vi "DE_Compare Population.vi"(10 "Population B":T2, 11 "Population A":T2) -> (2 "feasible?":bool, 3 "population comparison":T1 items=["A dominates B", "B dominates A", "Neither dominates", "A = B"])   [LabVIEW 2020, in "NI_AAL_GlobalOptimization.lvlib"]
uses:
  <vilib>/gmath/NI_AAL_GlobalOptimization.lvlib
  <vilib>/gmath/GlobalOptimization.llb/DE_Population.ctl
  <vilib>/gmath/GlobalOptimization.llb/DE_Population Comparison.ctl
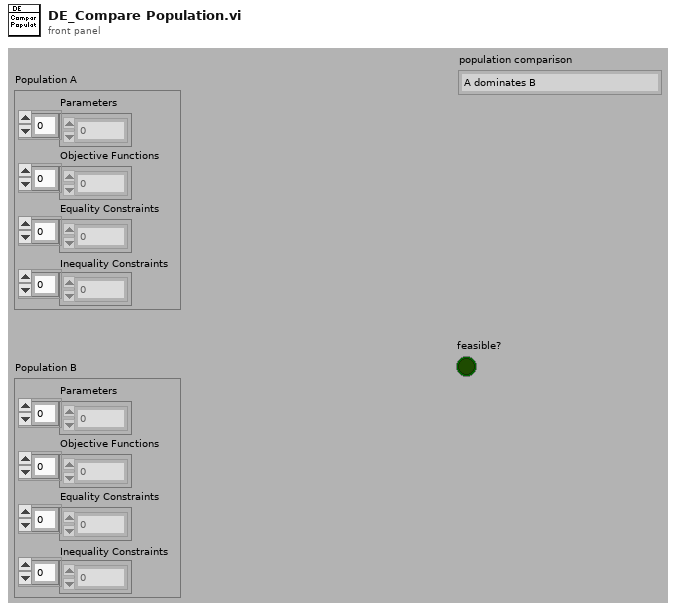
[diagram p1: front panel]
types:
  T1 = typedef "NI_AAL_GlobalOptimization.lvlib/DE_Population Comparison.ctl" = u16
  T2 = typedef "NI_AAL_GlobalOptimization.lvlib/DE_Population.ctl" = cluster{"Parameters":dbl[], "Objective Functions":dbl[], "Equality Constraints":dbl[], "Inequality Constraints":dbl[]}
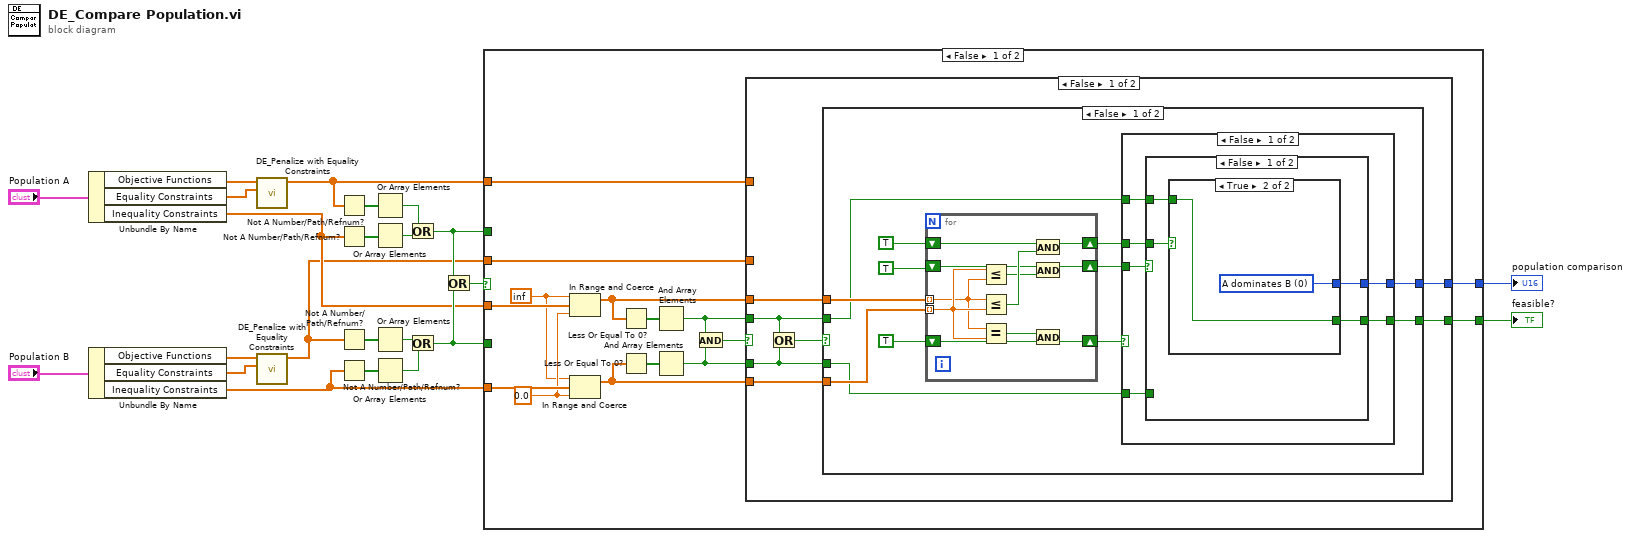
[diagram p0: block diagram]
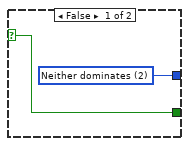
[diagram p2: hidden frame]
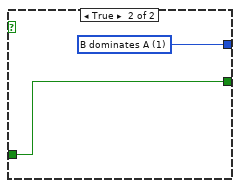
[diagram p3: hidden frame]
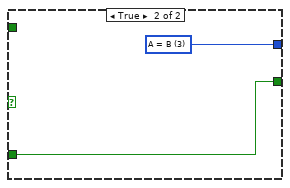
[diagram p4: hidden frame]
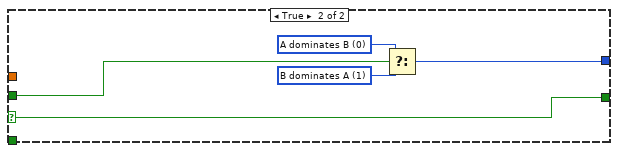
[diagram p5: hidden frame]
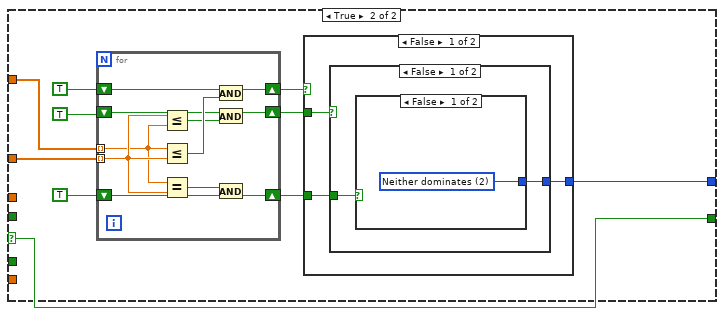
[diagram p6: hidden frame]
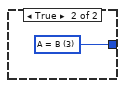
[diagram p7: hidden frame]
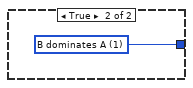
[diagram p8: hidden frame]
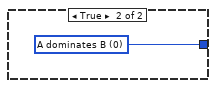
[diagram p9: hidden frame]
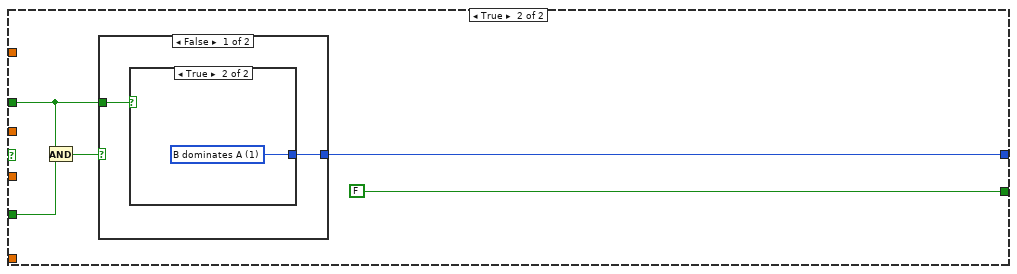
[diagram p10: hidden frame]
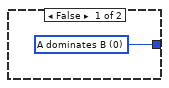
[diagram p11: hidden frame]
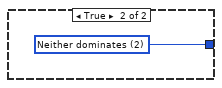
[diagram p12: hidden frame]
diagram:
  n1 = Unbundle By Name("Population A") -> ("Objective Functions"=w6:dbl[], "Equality Constraints"=w7:dbl[], "Inequality Constraints"=w8:dbl[])
  n2 = Unbundle By Name("Population B") -> ("Objective Functions"=w2:dbl[], "Equality Constraints"=w3:dbl[], "Inequality Constraints"=w4:dbl[])
  n3 = call <vilib>:"DE_Penalize with Equality Constraints.vi"("Equality Constraints"=w7, "Objective Functions In"=w6) -> ("Objective Functions Out"=w5:dbl[])  [unwired: 9 in]
  n4 = call <vilib>:"DE_Penalize with Equality Constraints.vi"("Equality Constraints"=w3, "Objective Functions In"=w2) -> ("Objective Functions Out"=w1:dbl[])  [unwired: 9 in]
  n5 = Not A Number/Path/Refnum?(number/path/refnum=w5) -> (NaN/Path/Refnum?=w19:bool[])
  n6 = Not A Number/Path/Refnum?(number/path/refnum=w8) -> (NaN/Path/Refnum?=w17:bool[])
  n7 = Not A Number/Path/Refnum?(number/path/refnum=w1) -> (NaN/Path/Refnum?=w18:bool[])
  n8 = Not A Number/Path/Refnum?(number/path/refnum=w4) -> (NaN/Path/Refnum?=w16:bool[])
  n9 = Or Array Elements(Boolean array=w19) -> (logical OR=w15:bool)
  n10 = Or Array Elements(Boolean array=w17) -> (logical OR=w14:bool)
  n11 = Or Array Elements(Boolean array=w18) -> (logical OR=w13:bool)
  n12 = Or Array Elements(Boolean array=w16) -> (logical OR=w12:bool)
  n13 = Or(x=w15, y=w14) -> (x .or. y?=w11:bool)
  n14 = Or(x=w13, y=w12) -> (x .or. y?=w10:bool)
  n15 = Or(x=w11, y=w10) -> (x .or. y?=w9:bool)
  n16 = case shown="False" w9 {
    tunnel: [w37 w124] -> w20
    tunnel: w5 -> [w36 _]
    tunnel: w8 -> [w34 _]
    tunnel: w4 -> [w31 _]
    tunnel: w1 -> [w35 _]
    tunnel: w11 -> [_ w123]
    tunnel: w10 -> [_ w126]
    tunnel: [w28 FALSE] -> w21
    frame False {
      w24 = inf
      w25 = 0.0
      n17 = In Range and Coerce(upper limit=w24, x=w34, lower limit=w25) -> (coerced(x)=w27:dbl[])  [unwired: 1 out]
      n18 = In Range and Coerce(upper limit=w24, x=w31, lower limit=w25) -> (coerced(x)=w26:dbl[])  [unwired: 1 out]
      n19 = Less Or Equal To 0?(x=w27) -> (x <= 0?=w33:bool[])
      n20 = Less Or Equal To 0?(x=w26) -> (x <= 0?=w32:bool[])
      n21 = And Array Elements(Boolean array=w33) -> (logical AND=w30:bool)
      n22 = And Array Elements(Boolean array=w32) -> (logical AND=w29:bool)
      n23 = And(x=w30, y=w29) -> (x .and. y?=w38:bool)
      n24 = case shown="False" w38 {
        selector: w38 -> [_ w92]
        tunnel: [w42 w98] -> w37
        tunnel: w36 -> [_ w94]
        tunnel: w35 -> [_ w93]
        tunnel: w30 -> [w43 _]
        tunnel: w29 -> [w44 _]
        tunnel: w27 -> [w41 _]
        tunnel: w26 -> [w40 _]
        tunnel: [w39 w92] -> w28
        frame False {
          n25 = Or(x=w43, y=w44) -> (x .or. y?=w45:bool)
          n26 = case shown="False" w45 {
            selector: w45 -> [_ w91]
            tunnel: w44 -> [w47 _]
            tunnel: w43 -> [w48 w90]
            tunnel: [w53 w87] -> w42
            tunnel: w41 -> [w52 _]
            tunnel: w40 -> [w51 _]
            tunnel: [w46 w91] -> w39
            frame False {
              n27 = for {
                tunnel: w52 -> [w78] mode=indexing
                tunnel: w51 -> [w79] mode=indexing
                shift-right: [w85] -> w49
                shift-left: TRUE -> [w86]
                shift-right: [w82] -> w50
                shift-left: TRUE -> [w83]
                shift-right: [w77] -> w54
                shift-left: TRUE -> [w76]
                n28 = Less Or Equal?(x=w79, y=w78) -> (x <= y?=w80:bool)
                n29 = Less Or Equal?(x=w78, y=w79) -> (x <= y?=w81:bool)
                n30 = Equal?(x=w78, y=w79) -> (x = y?=w84:bool)
                n31 = And(x=w86, y=w81) -> (x .and. y?=w85:bool)
                n32 = And(x=w76, y=w80) -> (x .and. y?=w77:bool)
                n33 = And(x=w84, y=w83) -> (x .and. y?=w82:bool)
              }
              n34 = case shown="False" w50 {
                tunnel: [w62 w74] -> w53
                tunnel: w54 -> [w63 _]
                tunnel: w49 -> [w61 _]
                tunnel: w48 -> [w60 _]
                tunnel: w47 -> [w59 w75]
                tunnel: [w58 w75] -> w46
                frame False {
                  n35 = case shown="False" w63 {
                    tunnel: [w66 w72] -> w62
                    tunnel: w61 -> [w67 _]
                    tunnel: w60 -> [w65 _]
                    tunnel: w59 -> [_ w73]
                    tunnel: [w64 w73] -> w58
                    frame False {
                      n36 = case shown="True" w67 {
                        selector: w67 -> [w69 _]
                        tunnel: [w68 w70] -> w66
                        tunnel: w65 -> [_ w71]
                        tunnel: [w69 w71] -> w64
                        frame False {
                          w68 = T1 2 items=["A dominates B", "B dominates A", "Neither dominates", "A = B"] ("population comparison")
                        }
                        frame True {
                          w70 = T1 0 items=["A dominates B", "B dominates A", "Neither dominates", "A = B"] ("population comparison")
                        }
                      }
                    }
                    frame True {
                      w72 = T1 1 items=["A dominates B", "B dominates A", "Neither dominates", "A = B"] ("population comparison")
                    }
                  }
                }
                frame True {
                  w74 = T1 3 items=["A dominates B", "B dominates A", "Neither dominates", "A = B"] ("population comparison")
                }
              }
            }
            frame True {
              w88 = T1 1 items=["A dominates B", "B dominates A", "Neither dominates", "A = B"] ("population comparison")
              w89 = T1 0 items=["A dominates B", "B dominates A", "Neither dominates", "A = B"] ("population comparison")
              n37 = Select(t=w89, s=w90, f=w88) -> (s? t:f=w87:T1)
            }
          }
        }
        frame True {
          n38 = for {
            tunnel: w94 -> [w113] mode=indexing
            tunnel: w93 -> [w114] mode=indexing
            shift-right: [w120] -> w99
            shift-left: TRUE -> [w121]
            shift-right: [w117] -> w95
            shift-left: TRUE -> [w118]
            shift-right: [w112] -> w96
            shift-left: TRUE -> [w111]
            n39 = Less Or Equal?(x=w114, y=w113) -> (x <= y?=w115:bool)
            n40 = Less Or Equal?(x=w113, y=w114) -> (x <= y?=w116:bool)
            n41 = Equal?(x=w113, y=w114) -> (x = y?=w119:bool)
            n42 = And(x=w121, y=w116) -> (x .and. y?=w120:bool)
            n43 = And(x=w111, y=w115) -> (x .and. y?=w112:bool)
            n44 = And(x=w119, y=w118) -> (x .and. y?=w117:bool)
          }
          n45 = case shown="False" w99 {
            tunnel: [w103 w110] -> w98
            tunnel: w96 -> [w104 _]
            tunnel: w95 -> [w102 _]
            frame False {
              n46 = case shown="False" w104 {
                tunnel: [w105 w109] -> w103
                tunnel: w102 -> [w106 _]
                frame False {
                  n47 = case shown="False" w106 {
                    tunnel: [w107 w108] -> w105
                    frame False {
                      w107 = T1 2 items=["A dominates B", "B dominates A", "Neither dominates", "A = B"] ("population comparison")
                    }
                    frame True {
                      w108 = T1 3 items=["A dominates B", "B dominates A", "Neither dominates", "A = B"] ("population comparison")
                    }
                  }
                }
                frame True {
                  w109 = T1 1 items=["A dominates B", "B dominates A", "Neither dominates", "A = B"] ("population comparison")
                }
              }
            }
            frame True {
              w110 = T1 0 items=["A dominates B", "B dominates A", "Neither dominates", "A = B"] ("population comparison")
            }
          }
        }
      }
    }
    frame True {
      n48 = And(x=w123, y=w126) -> (x .and. y?=w125:bool)
      n49 = case shown="False" w125 {
        tunnel: [w127 w131] -> w124
        tunnel: w123 -> [w128 _]
        frame False {
          n50 = case shown="True" w128 {
            tunnel: [w129 w130] -> w127
            frame False {
              w129 = T1 0 items=["A dominates B", "B dominates A", "Neither dominates", "A = B"] ("population comparison")
            }
            frame True {
              w130 = T1 1 items=["A dominates B", "B dominates A", "Neither dominates", "A = B"] ("population comparison")
            }
          }
        }
        frame True {
          w131 = T1 2 items=["A dominates B", "B dominates A", "Neither dominates", "A = B"] ("population comparison")
        }
      }
    }
  }
  "feasible?" <- w21
  "population comparison" <- w20
